vi "cluster test.vi"(11 "Controls[]":refnum<vi>[](array[refnum])) -> (0 "Dev groups (numbers)":string[](array[string]), 1 "Device controles":refnum<vi>[](array[refnum]), 2 "variable dev numbers":string[](array[string]), 3 "Caller variable names":string[](array[string]), 4 "Device Names":string[](array[string]), 5 "Enum controls":refnum<vi>[](array[refnum]), 6 "GUI Controls":refnum<vi>[](array[refnum]), 7 "Enable Subscribe":bool[](array[boolean]))   [LabVIEW 2020]
uses:
  <vilib>/Utility/VariantDataType/Type.ctl
  <vilib>/Utility/VariantDataType/VariantType.lvlib
panel:
  in  "Tab Control":enum32{"Page 1", "Page 2", "Page 3"}(tab)
  out "Variable Names":string[](array[string])
  out "Enable":bool[](array[boolean])
  out "Controls[] 2":refnum<vi>[](array[refnum])
  out "Name":string[](array[string])
  out "Data Type":T1[](array[typedef])
  out "Array 2":string[](array[string])
  out "Enums":string[](array[string])
  out "Number controls":i32
  out "error out 2":errorcluster
  out "Label.Text":string
  out "error out":errorcluster
  in  "error in":errorcluster
  out "Array":string[](array[string])
  out "Device number":string[](array[string])
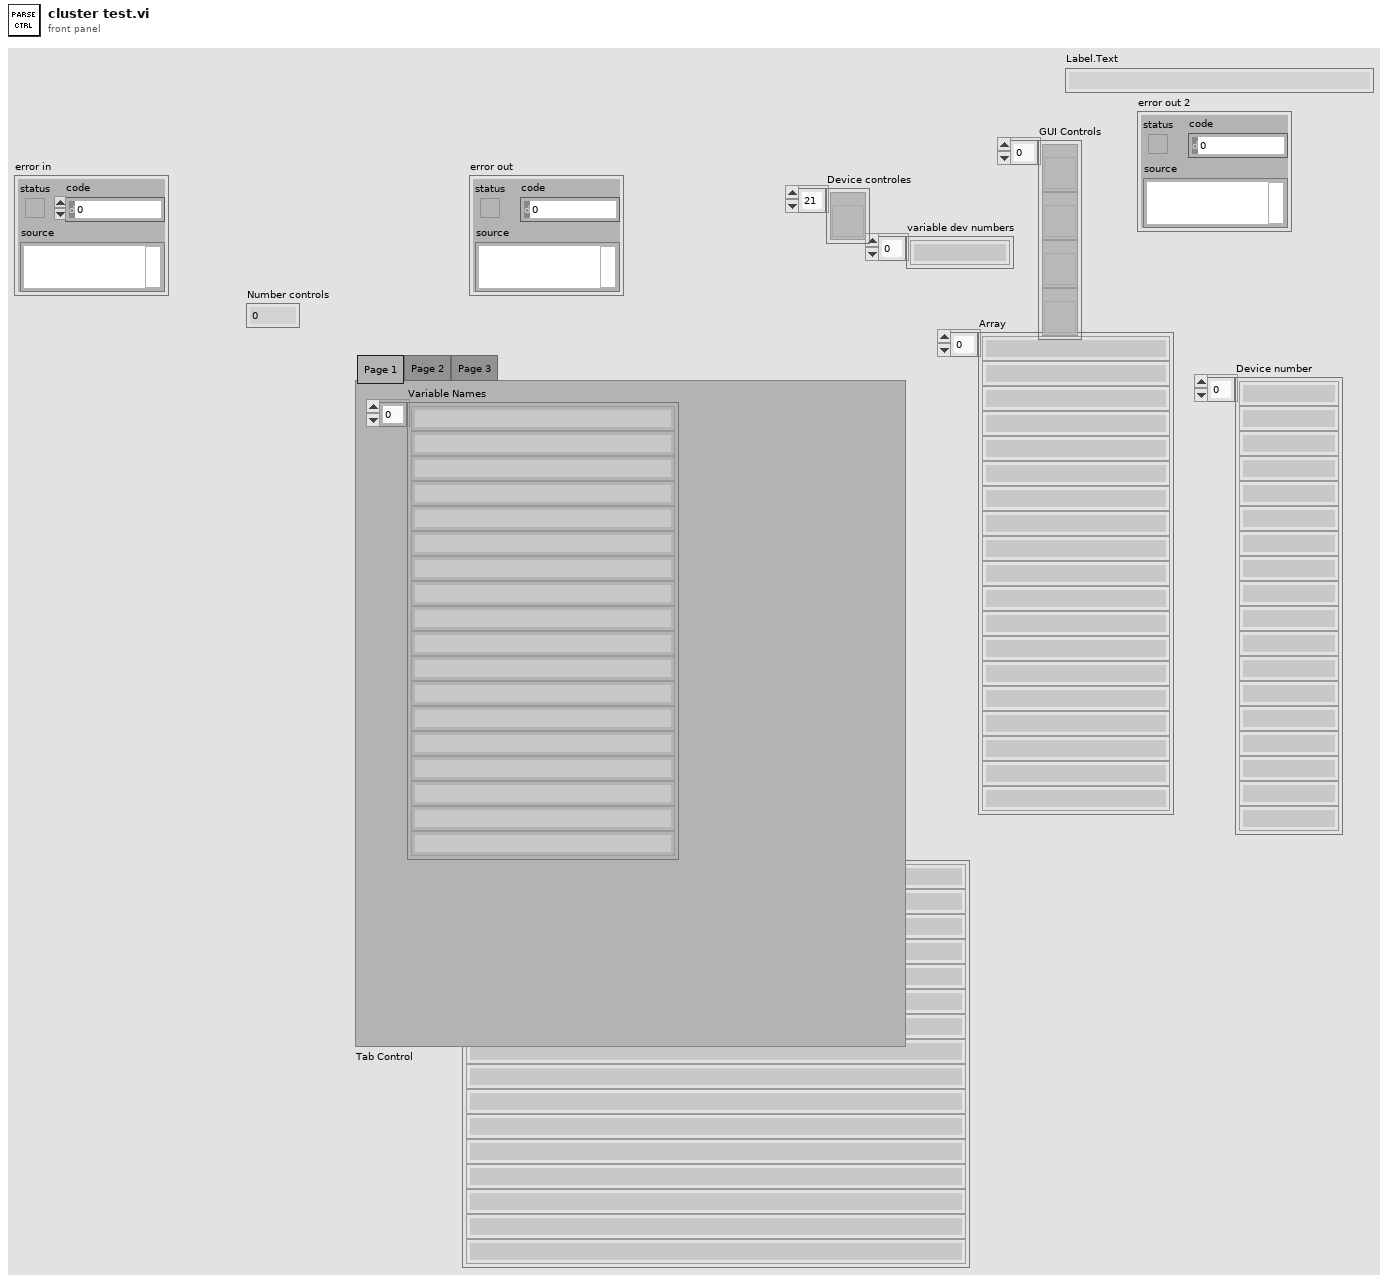
[diagram p1: front panel]
types:
  T1 = typedef "VariantType.lvlib/Type.ctl" = enum8{"Invalid Type", "Void", "I8", "I16", "I32", "I64", "U8", "U16", "U32", "U64", "Single Float", "Double Float", "Extended Float", "Single Complex", "Double Complex", "Extended Complex", "Enum U8", "Enum U16", "Enum U32", "Enum U64", "Single Float With Unit", "Double Float With Unit", "Extended Float With Unit", "Single Complex with Unit", "Double Complex with Unit", "Extended Complex with Unit", "Boolean", "String", "Path", "Picture", "Tag", "Array", "Cluster", "Variant", "LV Variant", "Waveform", "Timestamp", "Digital Waveform", "Digital Data", "ExpressData", "Refnum", "External Data", "VI", "Poly VI", "LabVIEW Class Instance", "Fixed Point"}
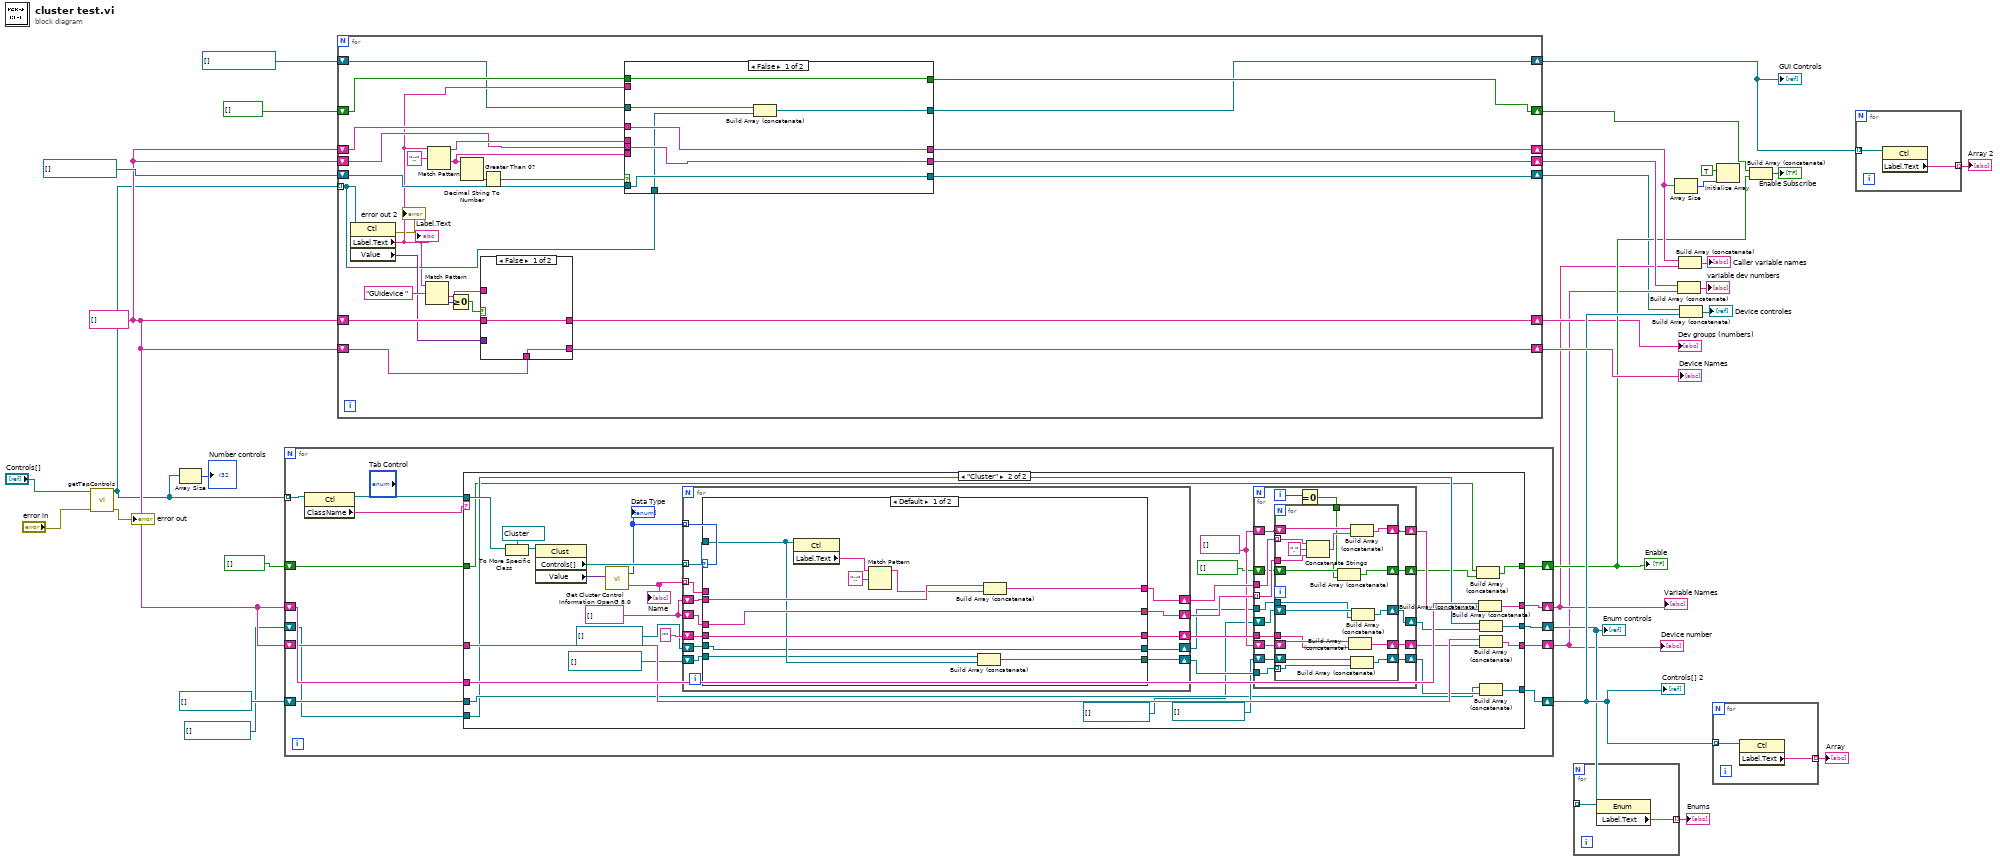
[diagram p0: block diagram]
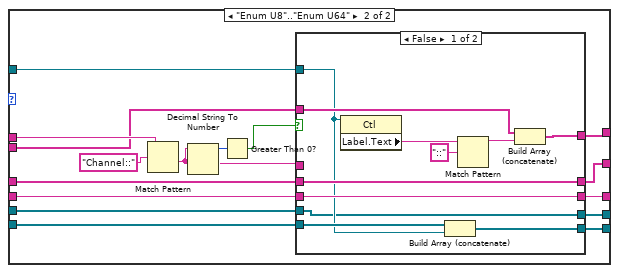
[diagram p3: hidden frame]
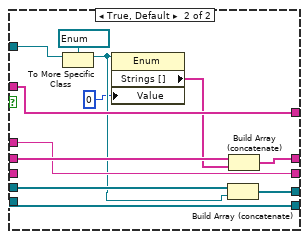
[diagram p4: hidden frame]
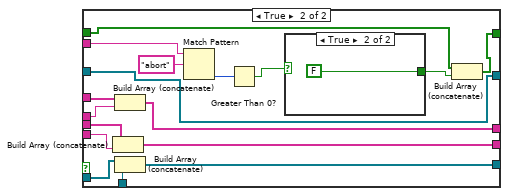
[diagram p5: hidden frame]
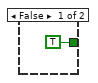
[diagram p6: hidden frame]
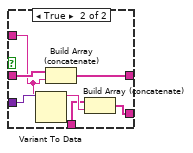
[diagram p7: hidden frame]
diagram:
  w31 = string[] [] ("Caller control labels")
  n1 = call "getTapControls.vi"("error in (no error)"="error in", "Controls[]"="Controls[]") -> ("error out"=→"error out":errorcluster, "controls out"=w2:refnum<vi>[])  [unwired: 8 in]
  n2 = Array Size(array=w2) -> (size(s)=→"Number controls":i32)
  n3 = for {
    shift-right: [w45] -> w9
    shift-left: w31 -> [w46]
    tunnel: w2 -> [w44] mode=indexing
    shift-right: [w41] -> w28
    shift-left: refnum<vi>[] [] ("Controls[]") -> [w42]
    shift-right: [w40] -> w8
    shift-left: w31 -> [w39]
    shift-right: [w38] -> w25
    shift-left: refnum<vi>[] [] ("Controls[]") -> [w37]
    shift-right: [w36] -> w19
    shift-left: bool[] [] ("Caller control labels") -> [w35]
    n4 = property class="Ctl"(reference=w44) -> (reference out=w43:refnum<vi>, "ClassName"=w34:string)  [unwired: 1 in, 1 out]
    n5 = case shown="\"Cluster\"" w34 {
      tunnel: [w51 w59] -> w45
      tunnel: w46 -> [w51 w78]
      tunnel: w43 -> [_ w74]
      tunnel: [w50 w64] -> w41
      tunnel: w42 -> [w50 w65]
      tunnel: [w49 w69] -> w40
      tunnel: w39 -> [w49 w71]
      tunnel: [w48 w57] -> w38
      tunnel: w37 -> [w48 w56]
      tunnel: [w47 w54] -> w36
      tunnel: w35 -> [w47 w52]
      frame "False", Default {
      }
      frame "Cluster" {
        w72 = string[] [] ("Caller control labels")
        w77 = string[] [] ("Caller control labels")
        n6 = To More Specific Class(target class=refnum<vi> refnum ("TESTITEM"), reference=w74) -> (specific class reference=w85:refnum<vi>)  [unwired: 1 in, 1 out]
        n7 = property class="Clust"(reference=w85) -> ("Controls[]"=w82:refnum<vi>[], "Value"=w83:variant)  [unwired: 1 in, 2 out]
        n8 = call "Get Cluster Control Information OpenG 8.0.vi"("Variant"=w83) -> ("Name"=w86:string[], "Data Type"=w81:T1[])  [unwired: 1 in]
        "Data Type" <- w81
        "Name" <- w86
        n9 = for {
          tunnel: w81 -> [w134] mode=indexing
          tunnel: w86 -> [w133] mode=indexing
          tunnel: w82 -> [w132] mode=indexing
          shift-right: [w130] -> w80
          shift-left: w77 -> [w131]
          shift-right: [w128] -> w76
          shift-left: w77 -> [w129]
          shift-right: [w126] -> w73
          shift-left: "" ("Label.Text") -> [w127]
          shift-right: [w124] -> w68
          shift-left: refnum<vi>[] [] ("Controls[]") -> [w125]
          shift-right: [w123] -> w62
          shift-left: refnum<vi>[] [] ("Controls[]") -> [w122]
          n10 = case shown="Default" w134 {
            tunnel: w133 -> [_ w160]
            tunnel: w132 -> [w141 w159]
            tunnel: w131 -> [w145 w155]
            tunnel: [w143 w156] -> w128
            tunnel: [w144 w154] -> w130
            tunnel: w129 -> [w143 w146]
            tunnel: w127 -> [w142 w151]
            tunnel: [w142 w152] -> w126
            tunnel: w125 -> [w140 w150]
            tunnel: [w139 w149] -> w124
            tunnel: [w135 w148] -> w123
            tunnel: w122 -> [w135 w147]
            frame Default {
              n11 = property class="Ctl"(reference=w141) -> ("Label.Text"=w137:string)  [unwired: 1 in, 2 out]
              n12 = Match Pattern(string=w137, regular expression="::") -> (before substring=w136:string)  [unwired: 1 in, 3 out]
              n13 = Build Array (concatenate)(w140, w141) -> (w139:refnum<vi>[])
              n14 = Build Array (concatenate)(w145, w136) -> (w144:string[])
            }
            frame "Enum U8".."Enum U64" {
              n15 = Match Pattern(string=w160, regular expression="Channel::") -> (after substring=w153:string)  [unwired: 1 in, 3 out]
              n16 = Decimal String To Number(string=w153) -> (number=w158:i32)  [unwired: 2 in, 1 out]
              n17 = Greater Than 0?(x=w158) -> (x > 0?=w157:bool)
              n18 = case shown="False" w157 {
                tunnel: w159 -> [w167 w183]
                tunnel: [w170 w179] -> w156
                tunnel: w155 -> [w172 w182]
                tunnel: [w171 w182] -> w154
                tunnel: w146 -> [w170 w181]
                tunnel: w153 -> [_ w178]
                tunnel: [w169 w178] -> w152
                tunnel: w151 -> [w169 _]
                tunnel: w150 -> [w168 w177]
                tunnel: [w166 w177] -> w149
                tunnel: [w162 w176] -> w148
                tunnel: w147 -> [w162 w175]
                frame False {
                  n19 = property class="Ctl"(reference=w167) -> ("Label.Text"=w164:string)  [unwired: 1 in, 2 out]
                  n20 = Build Array (concatenate)(w168, w167) -> (w166:refnum<vi>[])
                  n21 = Match Pattern(string=w164, regular expression="::") -> (before substring=w163:string)  [unwired: 1 in, 3 out]
                  n22 = Build Array (concatenate)(w172, w163) -> (w171:string[])
                }
                frame True, Default {
                  n23 = To More Specific Class(target class=refnum<vi> refnum ("TESTITEM"), reference=w183) -> (specific class reference=w174:refnum<vi>)  [unwired: 1 in, 1 out]
                  n24 = property class="Enum"(reference=w174, "Value"=0) -> ("Strings []"=w180:string[])  [unwired: 1 in, 2 out]
                  n25 = Build Array (concatenate)(w175, w174) -> (w176:refnum<vi>[])
                  n26 = Build Array (concatenate)(w181, w180) -> (w179:string[])
                }
              }
            }
          }
        }
        n27 = for {
          tunnel: w76 -> [w103] mode=indexing
          tunnel: w80 -> [w102]
          shift-right: [w100] -> w79
          shift-left: w72 -> [w101]
          tunnel: w73 -> [w99]
          shift-right: [w97] -> w70
          shift-left: w72 -> [w98]
          tunnel: w68 -> [w96]
          shift-right: [w94] -> w66
          shift-left: refnum<vi>[] [] ("Controls[]") -> [w95]
          tunnel: w62 -> [w92]
          shift-right: [w91] -> w58
          shift-left: refnum<vi>[] [] ("Controls[]") -> [w93]
          shift-right: [w89] -> w53
          shift-left: bool[] [] ("Caller control labels") -> [w90]
          i -> [w88]
          n28 = Equal To 0?(x=w88) -> (x = 0?=w87:bool)
          n29 = for {
            tunnel: w103 -> [w115]
            tunnel: w102 -> [w114] mode=indexing
            shift-right: [w120] -> w100
            shift-left: w101 -> [w121]
            tunnel: w99 -> [w113]
            shift-right: [w118] -> w97
            shift-left: w98 -> [w119]
            tunnel: w96 -> [w109] mode=indexing
            shift-right: [w117] -> w94
            shift-left: w95 -> [w116]
            shift-right: [w111] -> w91
            shift-left: w93 -> [w112]
            tunnel: w92 -> [w110]
            shift-right: [w105] -> w89
            shift-left: w90 -> [w106]
            tunnel: w87 -> [w104]
            n30 = Concatenate Strings(w114, "." ("string"), w115) -> (w107:string)
            n31 = Build Array (concatenate)(w106, w104) -> (w105:bool[])
            n32 = Build Array (concatenate)(w119, w113) -> (w118:string[])
            n33 = Build Array (concatenate)(w121, w107) -> (w120:string[])
            n34 = Build Array (concatenate)(w116, w109) -> (w117:refnum<vi>[])
            n35 = Build Array (concatenate)(w112, w110) -> (w111:refnum<vi>[])
          }
        }
        n36 = Build Array (concatenate)(w52, w53) -> (w54:bool[])
        n37 = Build Array (concatenate)(w78, w79) -> (w59:string[])
        n38 = Build Array (concatenate)(w56, w58) -> (w57:refnum<vi>[])
        n39 = Build Array (concatenate)(w71, w70) -> (w69:string[])
        n40 = Build Array (concatenate)(w65, w66) -> (w64:refnum<vi>[])
      }
    }
  }
  "Variable Names" <- w9
  "Controls[] 2" <- w28
  "Device number" <- w8
  "Enum controls" <- w25
  "Enable" <- w19
  n41 = for {
    tunnel: w2 -> [w191] mode=indexing
    shift-right: [w208] -> w10
    shift-left: w31 -> [w209]
    shift-right: [w202] -> w29
    shift-left: w31 -> [w203]
    shift-right: [w198] -> w20
    shift-left: w31 -> [w197]
    shift-right: [w194] -> w30
    shift-left: w31 -> [w195]
    shift-right: [w192] -> w5
    shift-left: refnum<vi>[] [] ("Controls[]") -> [w193]
    shift-right: [w188] -> w16
    shift-left: bool[] [] -> [w190]
    shift-right: [w187] -> w6
    shift-left: refnum<vi>[] [] -> [w186]
    n42 = property class="Ctl"(reference=w191) -> (error out=→"error out 2":errorcluster, "Label.Text"=w189:string, "Value"=w204:variant)  [unwired: 1 in, 1 out]
    "Label.Text" <- w189
    n43 = Match Pattern(string=w189, regular expression="GUIdevice " ("search string/char (-)")) -> (after substring=w205:string, offset past match=w206:i32)  [unwired: 1 in, 2 out]
    n44 = Match Pattern(string=w189, regular expression="::") -> (before substring=w196:string, after substring=w199:string)  [unwired: 1 in, 2 out]
    n45 = Greater Or Equal To 0?(x=w206) -> (x >= 0?=w210:bool)
    n46 = Decimal String To Number(string=w199) -> (number=w201:i32)  [unwired: 2 in, 1 out]
    n47 = case shown="False" w210 {
      tunnel: w205 -> [_ w243]
      tunnel: w209 -> [w239 w246]
      tunnel: [w239 w245] -> w208
      tunnel: w204 -> [_ w244]
      tunnel: w203 -> [w238 w241]
      tunnel: [w238 w240] -> w202
      frame False {
      }
      frame True {
        n48 = Variant To Data(type=w243, Variant=w244) -> (data=w242:string)  [unwired: 1 in, 1 out]
        n49 = Build Array (concatenate)(w246, w243) -> (w245:string[])
        n50 = Build Array (concatenate)(w241, w242) -> (w240:string[])
      }
    }
    n51 = Greater Than 0?(x=w201) -> (x > 0?=w200:bool)
    n52 = case shown="False" w200 {
      tunnel: w199 -> [_ w235]
      tunnel: [w218 w234] -> w198
      tunnel: w197 -> [w218 w233]
      tunnel: w196 -> [_ w232]
      tunnel: w195 -> [w217 w231]
      tunnel: [w217 w230] -> w194
      tunnel: w193 -> [w216 w229]
      tunnel: [w216 w228] -> w192
      tunnel: w191 -> [w214 w227]
      tunnel: w190 -> [w215 w220]
      tunnel: [w215 w222] -> w188
      tunnel: w189 -> [_ w224]
      tunnel: [w213 w219] -> w187
      tunnel: w186 -> [w212 w219]
      frame False {
        n53 = Build Array (concatenate)(w212, w214) -> (w213:refnum<vi>[])
      }
      frame True {
        n54 = Build Array (concatenate)(w231, w235) -> (w230:string[])
        n55 = Build Array (concatenate)(w233, w232) -> (w234:string[])
        n56 = Build Array (concatenate)(w229, w227) -> (w228:refnum<vi>[])
        n57 = Match Pattern(string=w224, regular expression="abort") -> (offset past match=w226:i32)  [unwired: 1 in, 3 out]
        n58 = Greater Than 0?(x=w226) -> (x > 0?=w223:bool)
        n59 = case shown="True" w223 {
          tunnel: [TRUE FALSE] -> w221
          frame False {
          }
          frame True {
          }
        }
        n60 = Build Array (concatenate)(w220, w221) -> (w222:bool[])
      }
    }
  }
  "Dev groups (numbers)" <- w10
  "Device Names" <- w29
  "GUI Controls" <- w6
  n61 = for {
    tunnel: w25 -> [w248] mode=indexing
    tunnel: [w247] -> w24 mode=indexing
    n62 = property class="Enum"(reference=w248) -> ("Label.Text"=w247:string)  [unwired: 1 in, 2 out]
  }
  "Enums" <- w24
  n63 = Array Size(array=w20) -> (size(s)=w21:i32)
  n64 = Build Array (concatenate)(w30, w8) -> (→"variable dev numbers":string[])
  n65 = Build Array (concatenate)(w20, w9) -> (→"Caller variable names":string[])
  n66 = Build Array (concatenate)(w5, w28) -> (→"Device controles":refnum<vi>[])
  n67 = for {
    tunnel: w28 -> [w250] mode=indexing
    tunnel: [w249] -> w27 mode=indexing
    n68 = property class="Ctl"(reference=w250) -> ("Label.Text"=w249:string)  [unwired: 1 in, 2 out]
  }
  "Array" <- w27
  n69 = Initialize Array(TRUE, w21) -> ()  [unwired: 1 out]
  n70 = Build Array (concatenate)(w16, w19) -> (→"Enable Subscribe":bool[])
  n71 = for {
    tunnel: w6 -> [w252] mode=indexing
    tunnel: [w251] -> w14 mode=indexing
    n72 = property class="Ctl"(reference=w252) -> ("Label.Text"=w251:string)  [unwired: 1 in, 2 out]
  }
  "Array 2" <- w14
